vi "Execute Periodic Task.vi"(8 "error in":errorcluster, 11 "GUI Facade in":refnum<class "GUI Facade.lvclass">) -> (0 "error out":errorcluster, 3 "GUI Facade out":refnum<class "GUI Facade.lvclass">)   [LabVIEW 2018, in "GUI Facade.lvclass"]
doc: "Execute operations for facade on a periodic basis. These operations might be:\n* Checking for current data\n* Writing to files\n\netc, etc..."
uses:
  GUI Facade.lvclass
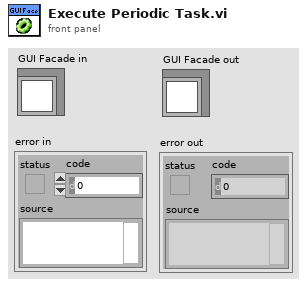
[diagram p1: front panel]
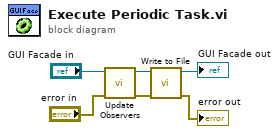
[diagram p0: block diagram]
diagram:
  n1 = call "Update Observers.vi"("error in"="error in", "GUI Facade in"="GUI Facade in") -> ("error out"=w3:errorcluster, "GUI Facade out"=w4:refnum<class "GUI Facade.lvclass">)  [unwired: 8 in]
  n2 = call-dynamic "Write to File.vi"("error in"=w3, "GUI Facade in"=w4) -> ("error out"=→"error out":errorcluster, "GUI Facade out"=→"GUI Facade out":refnum<class "GUI Facade.lvclass">)  [unwired: 8 in]
